vi "_save_csv_phaseCAL_Ken.vi"(7 "NoteName":string="SingleCh_", 11 "array in":string[][](array[string])) -> ()   [LabVIEW 2023, in "JIO.lvlib"]
uses:
  JIO.lvlib
  <vilib>/Utility/file.llb/Write Delimited Spreadsheet (string).vi
panel:
  out "FileName":string
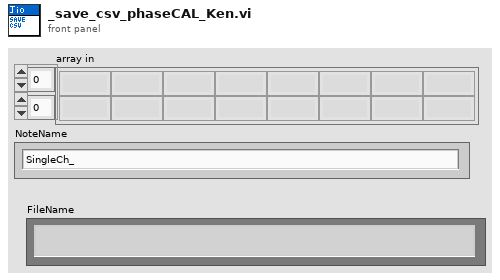
[diagram p1: front panel]
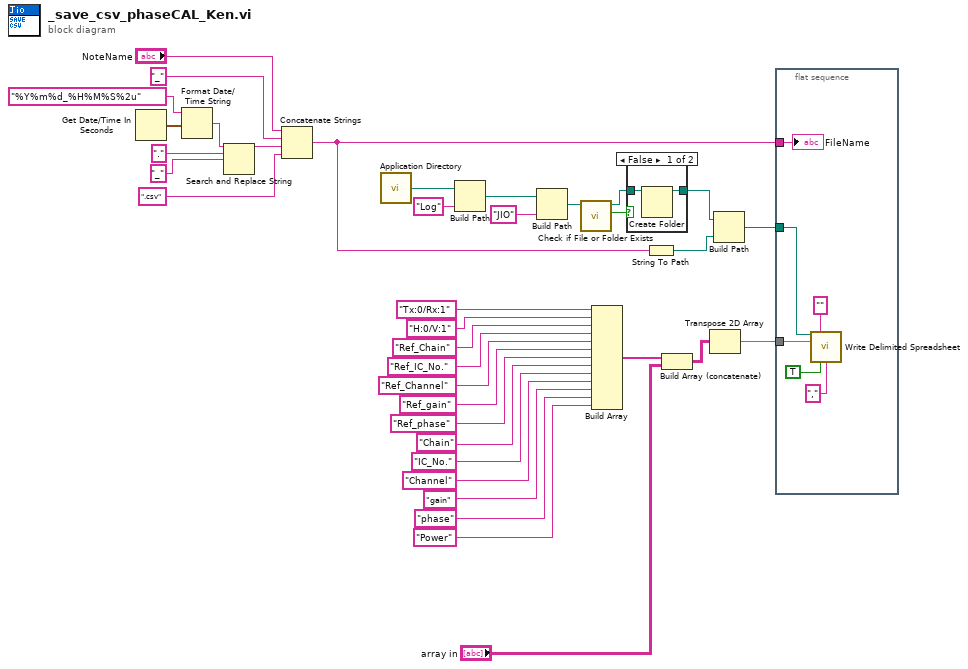
[diagram p0: block diagram]
diagram:
  n1 = Get Date/Time In Seconds() -> (seconds since 1Jan1904=w19:timestamp)
  n2 = Format Date/Time String(time format string (%c)="%Y%m%d_%H%M%S%2u", seconds (now)=w19) -> (date/time string=w17:string)  [unwired: 1 in]
  n3 = Search and Replace String(input string=w17, search string=".", replace string="_") -> (result string=w14:string)  [unwired: 5 in, 3 out]
  n4 = Concatenate Strings("NoteName", "_", w14, ".csv" ("delimiter (\\t)")) -> (w34:string)
  n5 = call <vilib>:"Application Directory.vi"() -> ("Application Directory"=w11:path)
  n6 = Build Path(base path=w11, name or relative path="Log") -> (appended path=w9:path)
  n7 = Build Path(base path=w9, name or relative path="JIO") -> (appended path=w8:path)
  n8 = call <vilib>:"Check if File or Folder Exists.vi"("path"=w8) -> ("file or folder exists?"=w33:bool, "dup path"=w32:path)  [unwired: 8 in, 1 out]
  n9 = Build Array("Tx:0/Rx:1", "H:0/V:1", "Ref_Chain", "Ref_IC_No.", "Ref_Channel", "Ref_gain", "Ref_phase", "Chain", "IC_No.", "Channel", "gain", "phase", "Power") -> (w22:string[])
  n10 = case shown="False" w33 {
    tunnel: w32 -> [w39 w40]
    tunnel: [w38 w40] -> w31
    frame False {
      n11 = Create Folder(path (use dialog)=w39) -> (created path=w38:path)  [unwired: 2 in, 2 out]
    }
    frame True {
    }
  }
  n12 = String To Path(string=w34) -> (path=w36:path)
  n13 = Build Array (concatenate)(w22, "array in") -> (w28:string[][])
  n14 = Transpose 2D Array(2D array=w28) -> (transposed array=w30:string[][])
  n15 = Build Path(base path=w31, name or relative path=w36) -> (appended path=w35:path)
  n16 = flat-sequence {
    tunnel: w35 -> [w45]
    tunnel: w34 -> [w43]
    tunnel: w30 -> [w41]
    frame #0 {
      n17 = call-poly <vilib>:"Write Delimited Spreadsheet.vi"("file path (dialog if empty)"=w45, "format (%s)"="" ("format (%.3f)"), "2D data"=w41, "transpose? (no:F)"=TRUE, "delimiter (\\t)"="," ("delimiter (\\t)")) -> ()  [unwired: 9 in, 2 out]
      "FileName" <- w43
    }
  }
